vi "main.vi"() -> ()   [LabVIEW 2021]
uses:
  typedefs/states.ctl
  typedefs/networkSettings.ctl
  typedefs/tcp_packet.ctl
  typedefs/tcp_cmd.ctl
  typedefs/tcp_states.ctl
  typedefs/commands.ctl
  <vilib>/ErrorRing/Error Ring.xnode
panel:
  out "tcp_packet":T1
  out "Console":string
  in  "Start":bool
  in  "Network settings":T4={"IP addr"="172.16.15.21", "port"=5000}
  out "State":T5
  in  "Exit":bool
  in  "Connect":bool
  # "typedef struct {\n    uint32_t cmd;\n    uint32_t state;\n    uint32_t num;\n    uint32_t len;\n    uint32_t err;\n    uint32_t data[];\n} tcp_packet_t;"
  # "typedef enum {\n    CMD_START = 0,\n    CMD_SOFTTRIG,\n    CMD_SETTSET,\n    CMD_SETTREAD,\n    CMD_TRANS_START,\n    CMD_TRANS_LEN,\n    CMD_TRANS_FINISH,\n} tcp_cmd_t;"
  # "typedef enum {\n    STATE_DISCONNECTED = 0,\n    STATE_IDLE,\n    STATE_WAITINGTRIG,\n    STATE_ACQUISITION,\n    STATE_DATARDY,\n    STATE_DATATRANS,\n    STATE_ERROR,\n} PhasemeterState_t;"
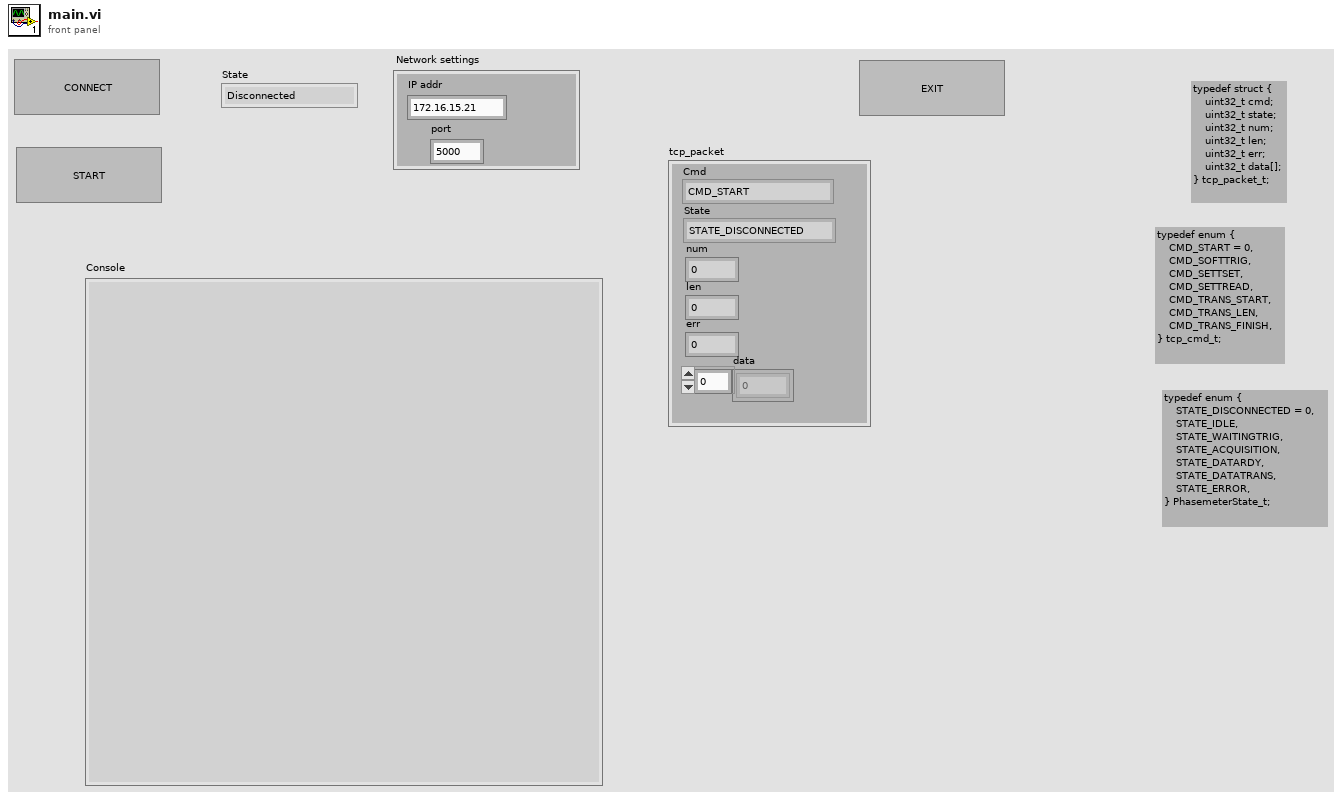
[diagram p1: front panel]
types:
  T1 = typedef "tcp_packet.ctl" = cluster{"Cmd":T2, "State":T3, "num":u32, "len":u32, "err":u32, "data":u32[]}
  T2 = typedef "tcp_cmd.ctl" = enum32{"CMD_START", "CMD_SOFTTRIG", "CMD_SETTSET", "CMD_SETTREAD", "CMD_TRANS_START", "CMD_TRANS_LEN", "CMD_TRANS_FINISH"}
  T3 = typedef "tcp_states.ctl" = enum32{"STATE_DISCONNECTED", "STATE_IDLE", "STAIT_WAITINGTRIG", "STATE_ACQUISITION", "STATE_DATARDY", "STATE_DATATRANS", "STATE_ERROR"}
  T4 = typedef "networkSettings.ctl" = cluster{"IP addr":string, "port":u16}
  T5 = typedef "states.ctl" = enum16{"Disconnected", "Idle", "Waiting for trigger", "Acquisition", "Data ready", "Data transfer", "Error"}
  T6 = typedef "commands.ctl" = enum16{"Exit", "Idle", "Connect", "Disconnect", "Start", "Finish", "Software trigger"}
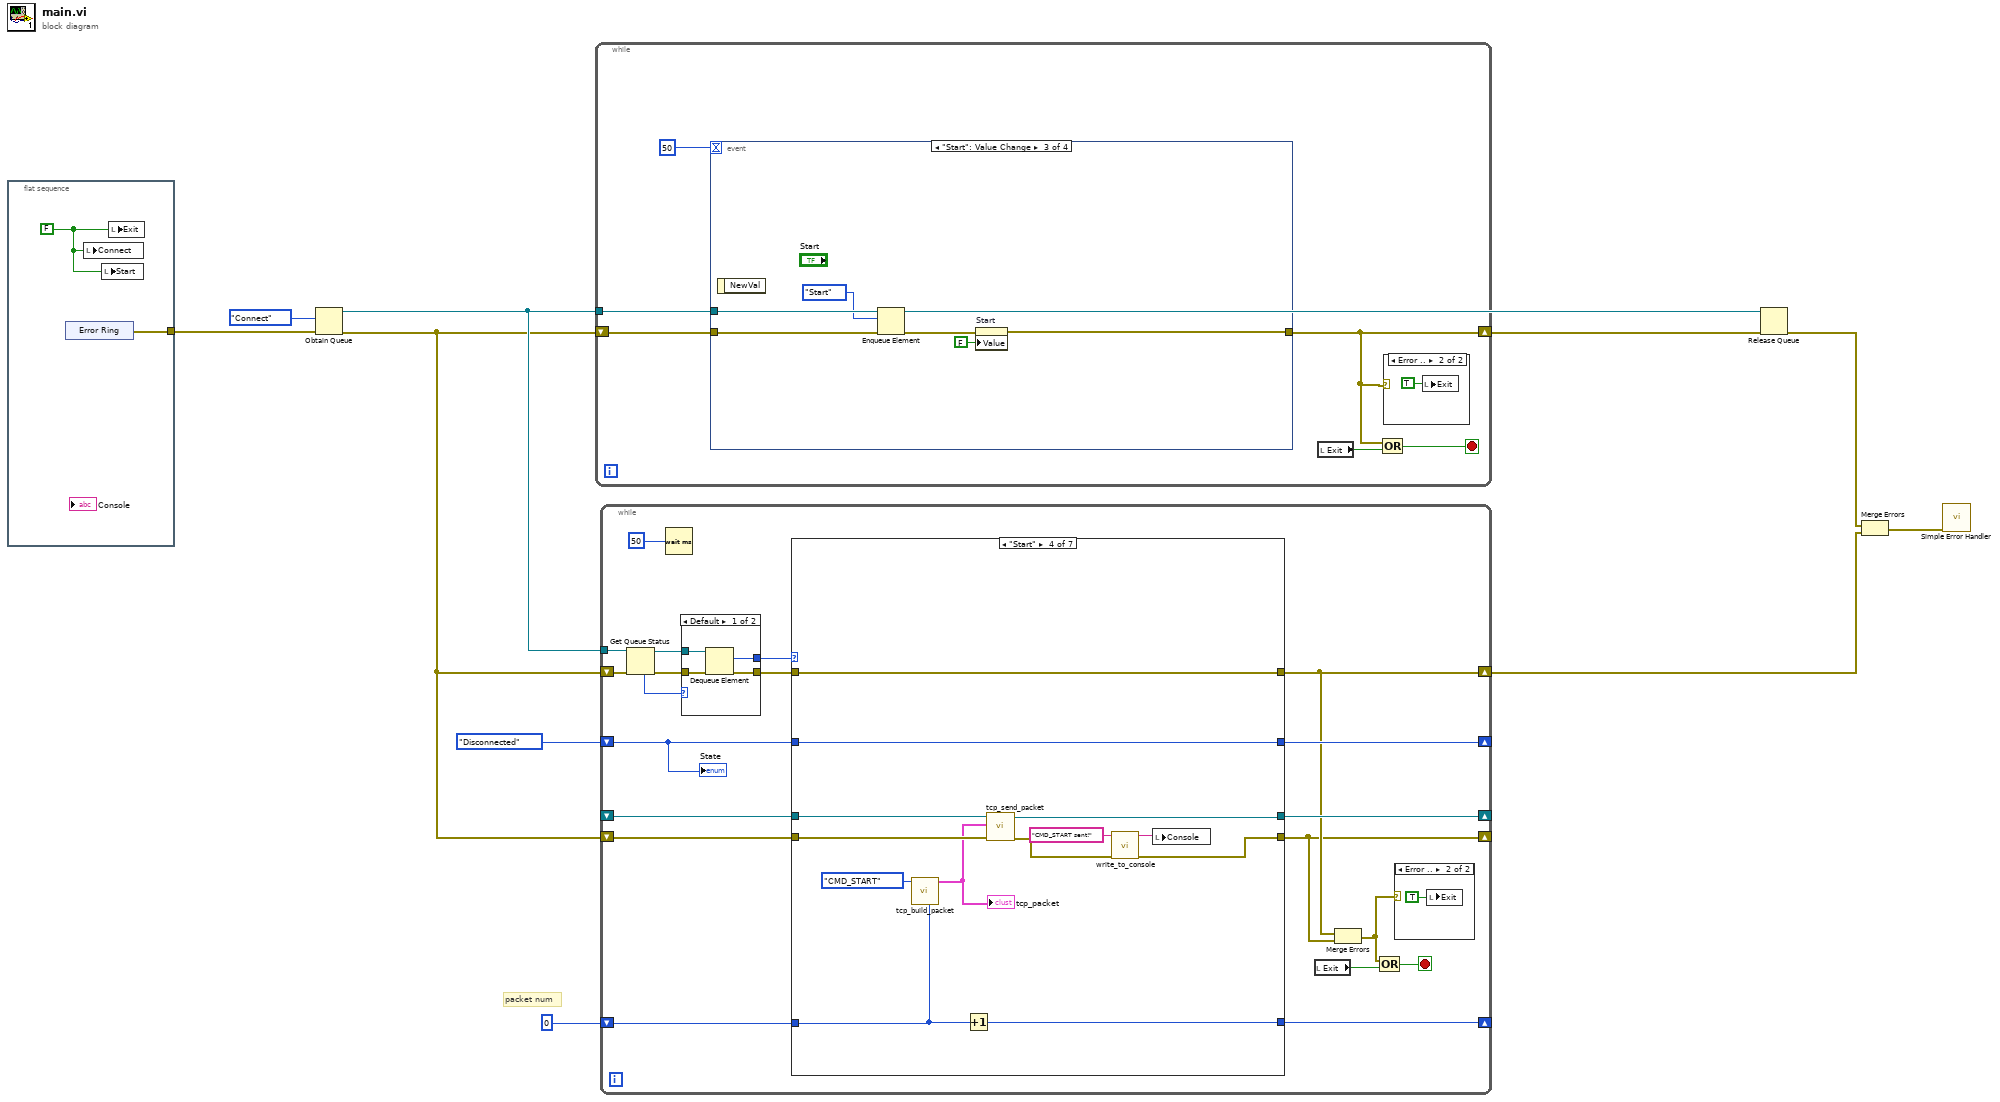
[diagram p0: block diagram]
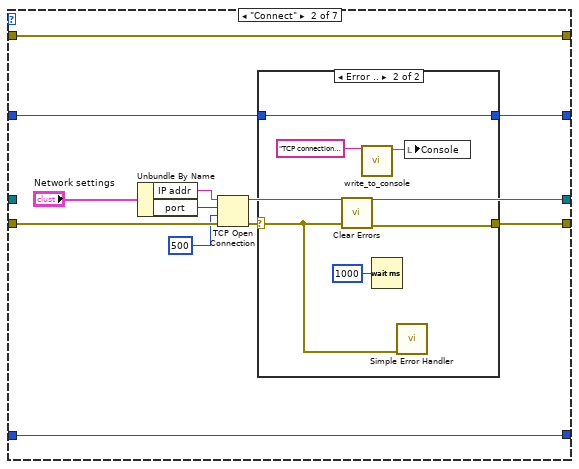
[diagram p4: hidden frame]
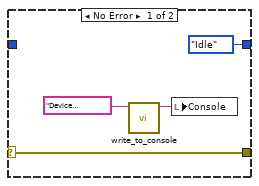
[diagram p5: hidden frame]
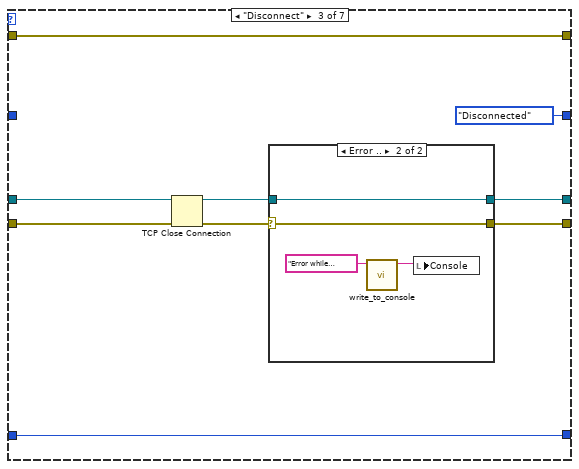
[diagram p6: hidden frame]
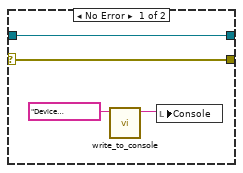
[diagram p7: hidden frame]
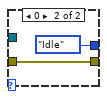
[diagram p11: hidden frame]
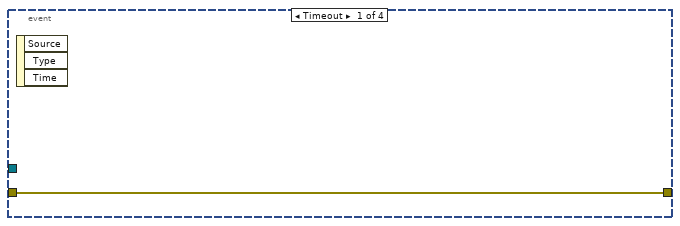
[diagram p13: hidden frame]
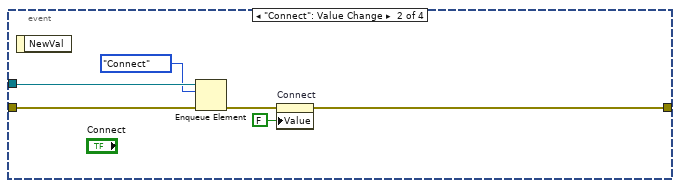
[diagram p14: hidden frame]
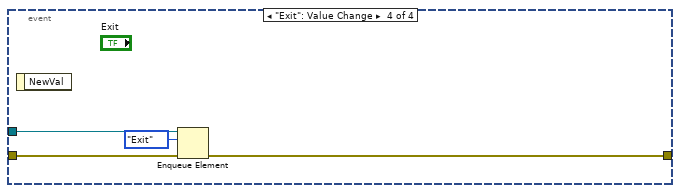
[diagram p15: hidden frame]
diagram:
  # "packet num"
  n1 = flat-sequence {
    tunnel: [w12] -> w3
    frame #0 {
      w11 = FALSE ("Exit")
      n2 = xnode "Error Ring"() -> ("error out"=w12:errorcluster)
      n3 = local write "Connect"(w11) -> ()
      n4 = local write "Start"(w11) -> ()
      n5 = local write "Exit"(w11) -> ()
    }
  }
  n6 = Obtain Queue(element data type=commands."Connect" ("Enum"), error in (no error)=w3) -> (queue out=w4:refnum<queue>, error out=w1:errorcluster)  [unwired: 3 in, 1 out]
  n7 = while {
    tunnel: w4 -> [w18]
    shift-right: [w14] -> w10
    shift-left: w1 -> [w17]
    stop <- w15 stop-if-true
    n8 = event shown="[2] \"Start\": Value Change" {
      selector: _ -> [_ _ _ _]
      dyn-events: _ -> [_ _ _ _]
      timeout: u32 50 ("milliseconds to wait") -> [_ _ _ _]
      tunnel: w18 -> [_ w27 w32 w35]
      tunnel: w17 -> [w21 w26 w33 w37]
      tunnel: [w21 w23 w30 w36] -> w14
      event Timeout {
        n9 = event-data() -> ()  [unwired: 1 in, 3 out]
      }
      event "Connect": Value Change {
        n10 = event-data() -> ()  [unwired: 1 in, 1 out]
        n11 = Enqueue Element(queue=w27, element=commands."Connect", error in (no error)=w26) -> (error out=w24:errorcluster)  [unwired: 1 in, 2 out]
        n12 = property on="Connect" class="Bool (strict)"(error in=w24, "Value"=FALSE ("Connect")) -> (error out=w23:errorcluster)  [unwired: 1 in, 1 out]
      }
      event "Start": Value Change {
        n13 = event-data() -> ()  [unwired: 1 in, 1 out]
        n14 = Enqueue Element(queue=w32, element=commands."Start", error in (no error)=w33) -> (error out=w31:errorcluster)  [unwired: 1 in, 2 out]
        n15 = property on="Start" class="Bool (strict)"(error in=w31, "Value"=FALSE ("Start")) -> (error out=w30:errorcluster)  [unwired: 1 in, 1 out]
      }
      event "Exit": Value Change {
        n16 = event-data() -> ()  [unwired: 1 in, 1 out]
        n17 = Enqueue Element(queue=w35, element=commands."Exit", error in (no error)=w37) -> (error out=w36:errorcluster)  [unwired: 1 in, 2 out]
      }
    }
    n18 = local read "Exit"() -> (w16:bool)
    n19 = Compound Arithmetic op=OR(w14, w16) -> (w15:bool)
    n20 = case shown="Error .." w14 {
      frame No Error {
      }
      frame Error {
        n21 = local write "Exit"(TRUE ("Exit")) -> ()
      }
    }
  }
  n22 = while {
    tunnel: w4 -> [w54]
    shift-right: [w43] -> w9
    shift-left: w1 -> [w53]
    shift-right: [w46] -> _
    shift-left: states."Disconnected" ("States") -> [w50]
    shift-right: [w42] -> _
    shift-left: w1 -> [w48]
    shift-right: [w47] -> _
    shift-left: _ -> [w40]
    shift-right: [w38] -> _
    shift-left: u32 0 -> [w39]
    stop <- w44 stop-if-true
    n23 = Get Queue Status(queue=w54, error in (no error)=w53) -> (queue out=w55:refnum<queue>, error out=w56:errorcluster, # elements in queue=w57:i32)  [unwired: 1 in, 5 out]
    n24 = Wait (ms)(milliseconds to wait=u32 50) -> ()  [unwired: 1 out]
    n25 = case shown="Default" w57 {
      tunnel: w56 -> [w134 w135]
      tunnel: w55 -> [w133 _]
      tunnel: [w132 w135] -> w49
      tunnel: [w131 commands."Idle" ("Enum")] -> w51
      frame Default {
        n26 = Dequeue Element(queue=w133, error in (no error)=w134) -> (element=w131:T6, error out=w132:errorcluster)  [unwired: 1 in, 2 out]
      }
      frame 0 {
      }
    }
    n27 = case shown="\"Start\"" w51 {
      tunnel: w50 -> [w63 w69 _ w115 w119 w124 w128]
      tunnel: w49 -> [w61 w67 w94 w114 w120 w125 w127]
      tunnel: w48 -> [w62 w75 w91 w109 w117 w122 w130]
      tunnel: [w62 w70 w88 w103 w117 w122 w130] -> w42
      tunnel: [w60 w74 w86 w108 w118 w123 w129] -> w47
      tunnel: [w63 w68 states."Disconnected" ("States") w115 w119 w124 w128] -> w46
      tunnel: [w61 w67 w94 w114 w120 w125 w127] -> w43
      tunnel: w40 -> [w60 _ w92 w110 w118 w123 w129]
      tunnel: w39 -> [w59 w65 w90 w113 w116 w121 w126]
      tunnel: [w59 w65 w90 w112 w116 w121 w126] -> w38
      frame "Idle", Default {
      }
      frame "Connect" {
        n28 = Unbundle By Name("Network settings") -> ("IP addr"=w72:string, "port"=w73:u16)
        n29 = TCP Open Connection(address=w72, remote port or service name=w73, timeout ms (60000)=500, error in (no error)=w75) -> (connection ID=w74:refnum<k5>, error out=w71:errorcluster)  [unwired: 1 in]
        n30 = case shown="Error .." w71 {
          selector: w71 -> [w79 w80]
          tunnel: [w79 w85] -> w70
          tunnel: w69 -> [_ w83]
          tunnel: [states."Idle" ("States") w83] -> w68
          frame No Error {
            n31 = call "write_to_console.vi"("input_str"="Device connected!") -> ("res_str"=w76:string)  [unwired: 9 in, 1 out]
            n32 = local write "Console"(w76) -> ()
          }
          frame Error {
            n33 = call <vilib>:"Clear Errors.vi"("error in (no error)"=w80) -> ("error out"=w85:errorcluster)  [unwired: 5 in, 1 out]
            n34 = call "write_to_console.vi"("input_str"="TCP connection error!") -> ("res_str"=w82:string)  [unwired: 9 in, 1 out]
            n35 = Wait (ms)(milliseconds to wait=u32 1000) -> ()  [unwired: 1 out]
            n36 = call <vilib>:"Simple Error Handler.vi"("error in (no error)"=w80) -> ()  [unwired: 4 in, 5 out]
            n37 = local write "Console"(w82) -> ()
          }
        }
      }
      frame "Disconnect" {
        n38 = TCP Close Connection(connection ID=w92, error in (no error)=w91) -> (connection ID out=w87:refnum<k5>, error out=w89:errorcluster)  [unwired: 1 in]
        n39 = case shown="Error .." w89 {
          selector: w89 -> [w98 w100]
          tunnel: [w98 w100] -> w88
          tunnel: w87 -> [w95 w99]
          tunnel: [w95 w99] -> w86
          frame No Error {
            n40 = call "write_to_console.vi"("input_str"="Device disconnected!") -> ("res_str"=w97:string)  [unwired: 9 in, 1 out]
            n41 = local write "Console"(w97) -> ()
          }
          frame Error {
            n42 = call "write_to_console.vi"("input_str"="Error while disconnecting!") -> ("res_str"=w102:string)  [unwired: 9 in, 1 out]
            n43 = local write "Console"(w102) -> ()
          }
        }
      }
      frame "Start" {
        n44 = call "tcp_build_packet.vi"("num"=w113, "Cmd"=tcp_cmd."CMD_START") -> ("tcp_packet"=w107:T1)  [unwired: 9 in]
        "tcp_packet" <- w107
        n45 = Increment(x=w113) -> (x+1=w112:u32)
        n46 = call "tcp_send_packet.vi"("error in (no error)"=w109, "tcp_packet"=w107, "TCP Network Connection in"=w110) -> ("error out"=w104:errorcluster, "TCP Network Connection out"=w108:refnum<k5>)  [unwired: 7 in]
        n47 = call "write_to_console.vi"("error in"=w104, "input_str"="CMD_START sent!") -> ("error out"=w103:errorcluster, "res_str"=w106:string)  [unwired: 8 in]
        n48 = local write "Console"(w106) -> ()
      }
      frame "Finish" {
      }
      frame "Software trigger" {
      }
      frame "Exit" {
      }
    }
    n49 = local read "Exit"() -> (w45:bool)
    n50 = Merge Errors(w43, w42) -> (w41:errorcluster)
    n51 = Compound Arithmetic op=OR(w41, w45) -> (w44:bool)
    n52 = case shown="Error .." w41 {
      frame No Error {
      }
      frame Error {
        n53 = local write "Exit"(TRUE ("Exit")) -> ()
      }
    }
    "State" <- w50
  }
  n54 = Release Queue(queue=w4, error in (no error)=w10) -> (error out=w8:errorcluster)  [unwired: 1 in, 2 out]
  n55 = Merge Errors(w8, w9) -> (w7:errorcluster)
  n56 = call <vilib>:"Simple Error Handler.vi"("error in (no error)"=w7) -> ()  [unwired: 4 in, 5 out]
